vi "注册机.vi"() -> ()   [LabVIEW 2014]
uses:
  <userlib>/_OpenG.lib/md5/md5.llb/MD5 Message Digest (Hexadecimal String)__ogtk.vi
panel:
  in  "天数":i32=30
  in  "授权类型":u16(ring) items=["试用版", "正式版"]
  in  "退出":bool
  in  "生成":bool
  out "license":string
  in  "机器码":string
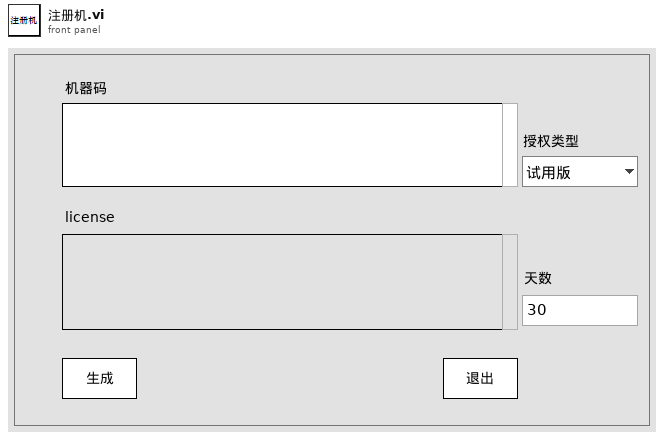
[diagram p1: front panel]
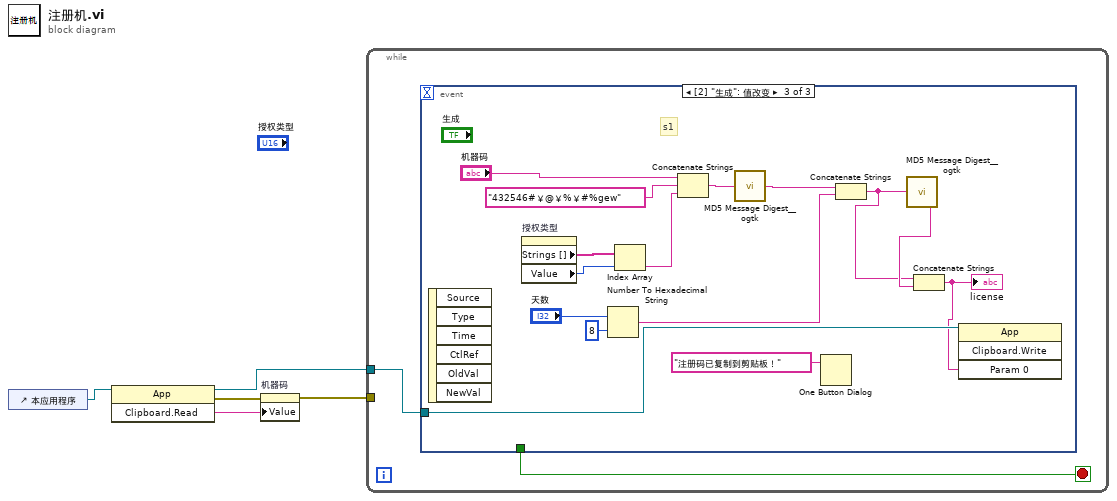
[diagram p0: block diagram]
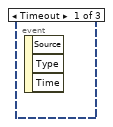
[diagram p2: hidden frame]
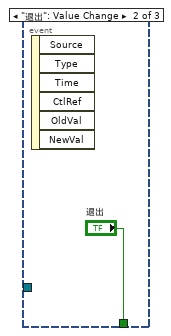
[diagram p3: hidden frame]
diagram:
  n1 = control-ref of="本应用程序"() -> (w5:refnum<vi>)
  n2 = invoke class="App" method="Clipboard.Read"(reference=w5) -> (reference out=w1:refnum<vi>, error out=w4:errorcluster, "Read Clipbrd"=w2:string)  [unwired: 2 in]
  n3 = property on="机器码" class="Str"(error in=w4, "Value"=w2) -> (error out=w3:errorcluster)  [unwired: 1 in, 1 out]
  n4 = while {
    tunnel: w3 -> [_]
    tunnel: w1 -> [w7]
    stop <- w6 stop-if-true
    n5 = event shown="[2] \"生成\": 值改变" {
      selector: _ -> [_ _ _]
      dyn-events: _ -> [_ _ _]
      timeout: _ -> [_ _ _]
      tunnel: w7 -> [_ _ w11]
      tunnel: [_ "退出" _] -> w6
      event Timeout {
        n6 = event-data() -> ()  [unwired: 1 in, 3 out]
      }
      event "退出": Value Change {
        n7 = event-data() -> ()  [unwired: 1 in, 6 out]
      }
      event "生成": Value Change {
        # "s1"
        n8 = event-data() -> ()  [unwired: 1 in, 6 out]
        n9 = property on="授权类型" class="Ring (严格)"() -> ("Strings []"=w21:string[], "Value"=w20:u16)  [unwired: 2 in, 2 out]
        n10 = Number To Hexadecimal String(1:i16 8 ("宽度(-)"), 2:"天数") -> (0:w14:string)
        n11 = Index Array(array=w21, index=w20) -> (element=w19:string)
        n12 = Concatenate Strings("机器码", "432546#￥@￥%￥#%gew", w19) -> (w18:string)
        n13 = call-poly <userlib>:"MD5 Message Digest__ogtk.vi"("Message"=w18) -> ("MD5 Message Digest"=w15:string)
        n14 = One Button Dialog(message="注册码已复制到剪贴板！" ("消息")) -> ()  [unwired: 1 in, 1 out]
        n15 = Concatenate Strings(w15, w14) -> (w12:string)
        n16 = call-poly <userlib>:"MD5 Message Digest__ogtk.vi"("Message"=w12) -> ("MD5 Message Digest"=w13:string)
        n17 = Concatenate Strings(w12, w13) -> (w10:string)
        "license" <- w10
        n18 = invoke class="App" method="Clipboard.Write"(reference=w11, "Param 0"=w10) -> ()  [unwired: 2 in, 4 out]
      }
    }
  }
